vi "Substract_Spectrum.vi"(0 "Substract Background":bool, 2 "spectrum":dbl[](array[numeric]), 3 "background spectrum":dbl[](array[numeric])) -> (8 "output spectrum":dbl[](array[numeric]))   [LabVIEW 2013]
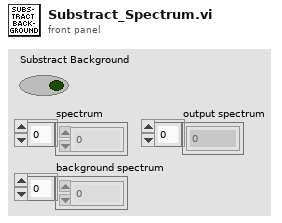
[diagram p1: front panel]
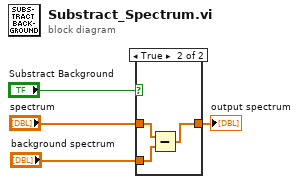
[diagram p0: block diagram]
diagram:
  n1 = case shown="True" "Substract Background" {
    tunnel: "background spectrum" -> [_ w7]
    tunnel: "spectrum" -> [w5 w8]
    tunnel: [w5 w6] -> w1
    frame False {
    }
    frame True {
      n2 = Subtract(x=w8, y=w7) -> (x-y=w6:dbl[])
    }
  }
  "output spectrum" <- w1
